vi "FirstDayMG.vi"() -> ()   [LabVIEW 2012]
panel:
  out "D":dbl
  in  "C":dbl(slide) scale=0.0..200.0
  out "N33DL3":dbl(knob) scale=0.0..200.0
  in  "stop":bool
  out "F":dbl
  in  "B":dbl(slide) scale=0.0..50.0
  in  "A":dbl(knob) scale=0.0..200.0
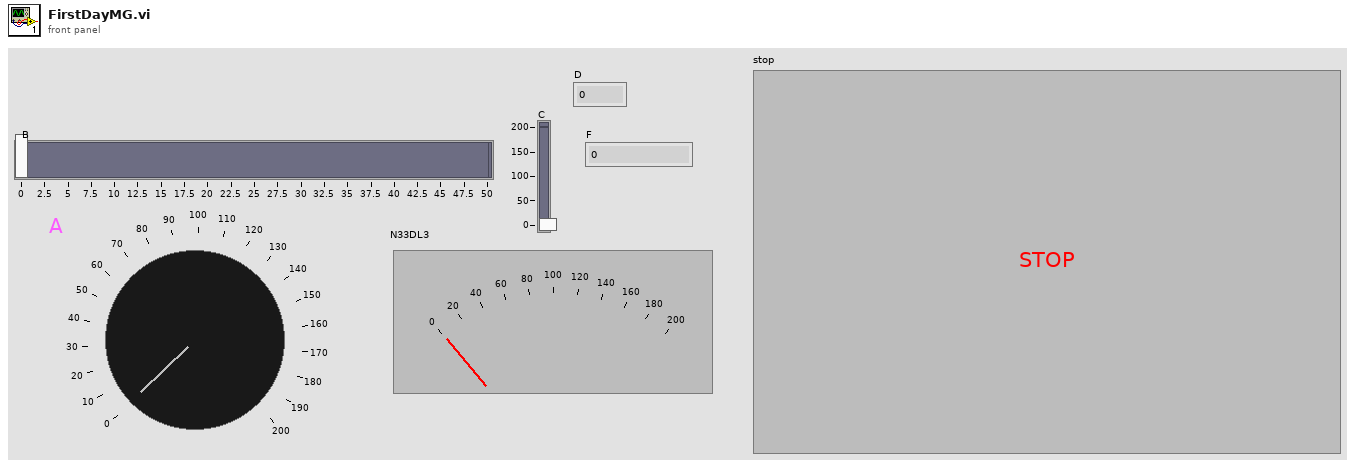
[diagram p1: front panel]
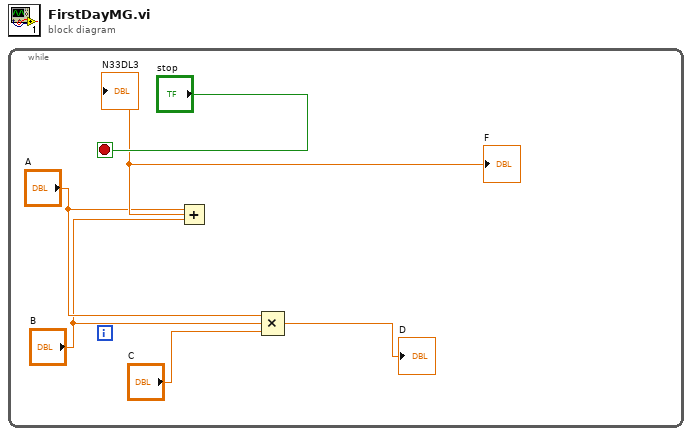
[diagram p0: block diagram]
diagram:
  n1 = while {
    stop <- "stop" stop-if-true
    n2 = Add(x="A", y="B") -> (x+y=→"F" →"N33DL3":dbl)
    n3 = Compound Arithmetic op=MULTIPLY("A", "B", "C") -> (→"D":dbl)
  }
